vi "Dynamic Launch Nested Actor.vi"(8 "error in (no error)":errorcluster, 11 "UI ActorTop in":refnum<class "MouseHandle.lvclass">) -> (0 "error out":errorcluster, 3 "UI ActorTop out":refnum<class "MouseHandle.lvclass">)   [LabVIEW 2021, in "MouseHandle.lvlib" / "MouseHandle.lvclass"]
doc: "Use Launch Nested Actor.vi to dynamic load child VI.\n2015-04-02 12:54:56\n蒋松\njiangsong@outlook.com"
uses:
  MouseHandle.lvclass
  MouseHandle.lvclass/MouseHandle.ctl
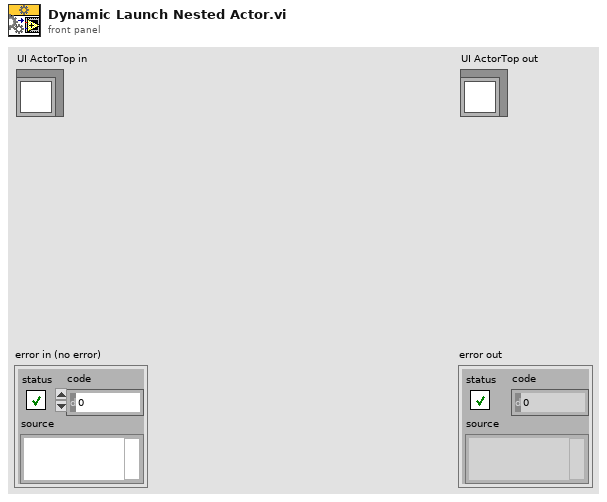
[diagram p1: front panel]
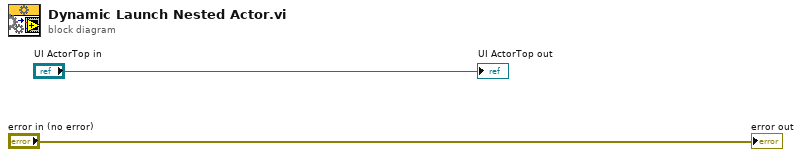
[diagram p0: block diagram]
diagram:
  "error out" <- "error in (no error)"
  "UI ActorTop out" <- "UI ActorTop in"
